vi "VPA QC Calibrate XDCRs.vi"(7 "DAQ Q":T1, 9 "DAQ Ref Cluster":T2, 10 "State Cluster":T4) -> (2 "State Cluster Out":T4)   [LabVIEW 2013]
uses:
  Controls/VPA QC State Data Cluster.ctl
  Controls/VPA QC General Cluster.ctl
  Controls/VPA QC State Enum.ctl
  Controls/VPA QC Bool Cluster.ctl
  Controls/VPA QC DAQ Ref Cluster.ctl
  Controls/VPA QC Scale Communication Settings DVR.ctl
  Controls/VPA QC Scale Communication Settings.ctl
  Controls/VPA QC DAQ Q.ctl
  Controls/VPA QC DAQ Cmd Enum.ctl
panel:
  out "Data Array":dbl[][](array[numeric])
  in  "Take 0 PSI":bool
  in  "Clear Data":bool
  out "Status":string
  out "Best Fit Y-Intercept":dbl format="%0.2f"
  out "Best Fit Slope":dbl format="%0.4f"
  in  "Ramp Down":bool
  in  "Stop Ramp":bool
  out "PcurB":dbl
  in  "Start Ramp":bool
  in  "Pressure Set Point":u32=100 min=100 max=10000
  in  "Open Outlet Valves":bool
  in  "Enterered New\n Volts Constant for B":dbl
  out "Estimated New Max\nVolts for B cylinder.":dbl
  out "PcurA":dbl
  out "A-B Graph":cluster{"X":dbl[], "Y":dbl[]}[](graph)
  in  "Cancel":bool
  in  "Save":bool
  # "Match Pressure Transducers"
  # "Step 1: Make sure the cylinders are initialized and cycled. \nStep 2: Open outlet valves and make sure the cylinders both read 0 psi (or within 1 psi of zero). If they don't zero the transducders."
  # "Step 3: Take a point at 0"
  # "Step 4: Make sure the external outlet valve is closed.\nStep 5. Set the pressue to match the transducers at (you can do this multiple times to see the best fit slope for multiple values.)"
  # "Step 6:"
  # "Monitor the pump. Make sure pump is idle and the external valve is closed. This program will control pressure in a method that bypasses normal procedure.  Turn the pump off if cylinders begin moving too quickly."
  # "Step 7: Determine new volts to use for B side. After ramping pressure down, use terminal to input new max volts for the B cylinder and save the value here for reference."
  # "Suggested\nB Volts"
  # "PcurA"
  # "PcurB"
  # "Dif."
  # "Assembly Checklist"
  # "Assembly Checklist"
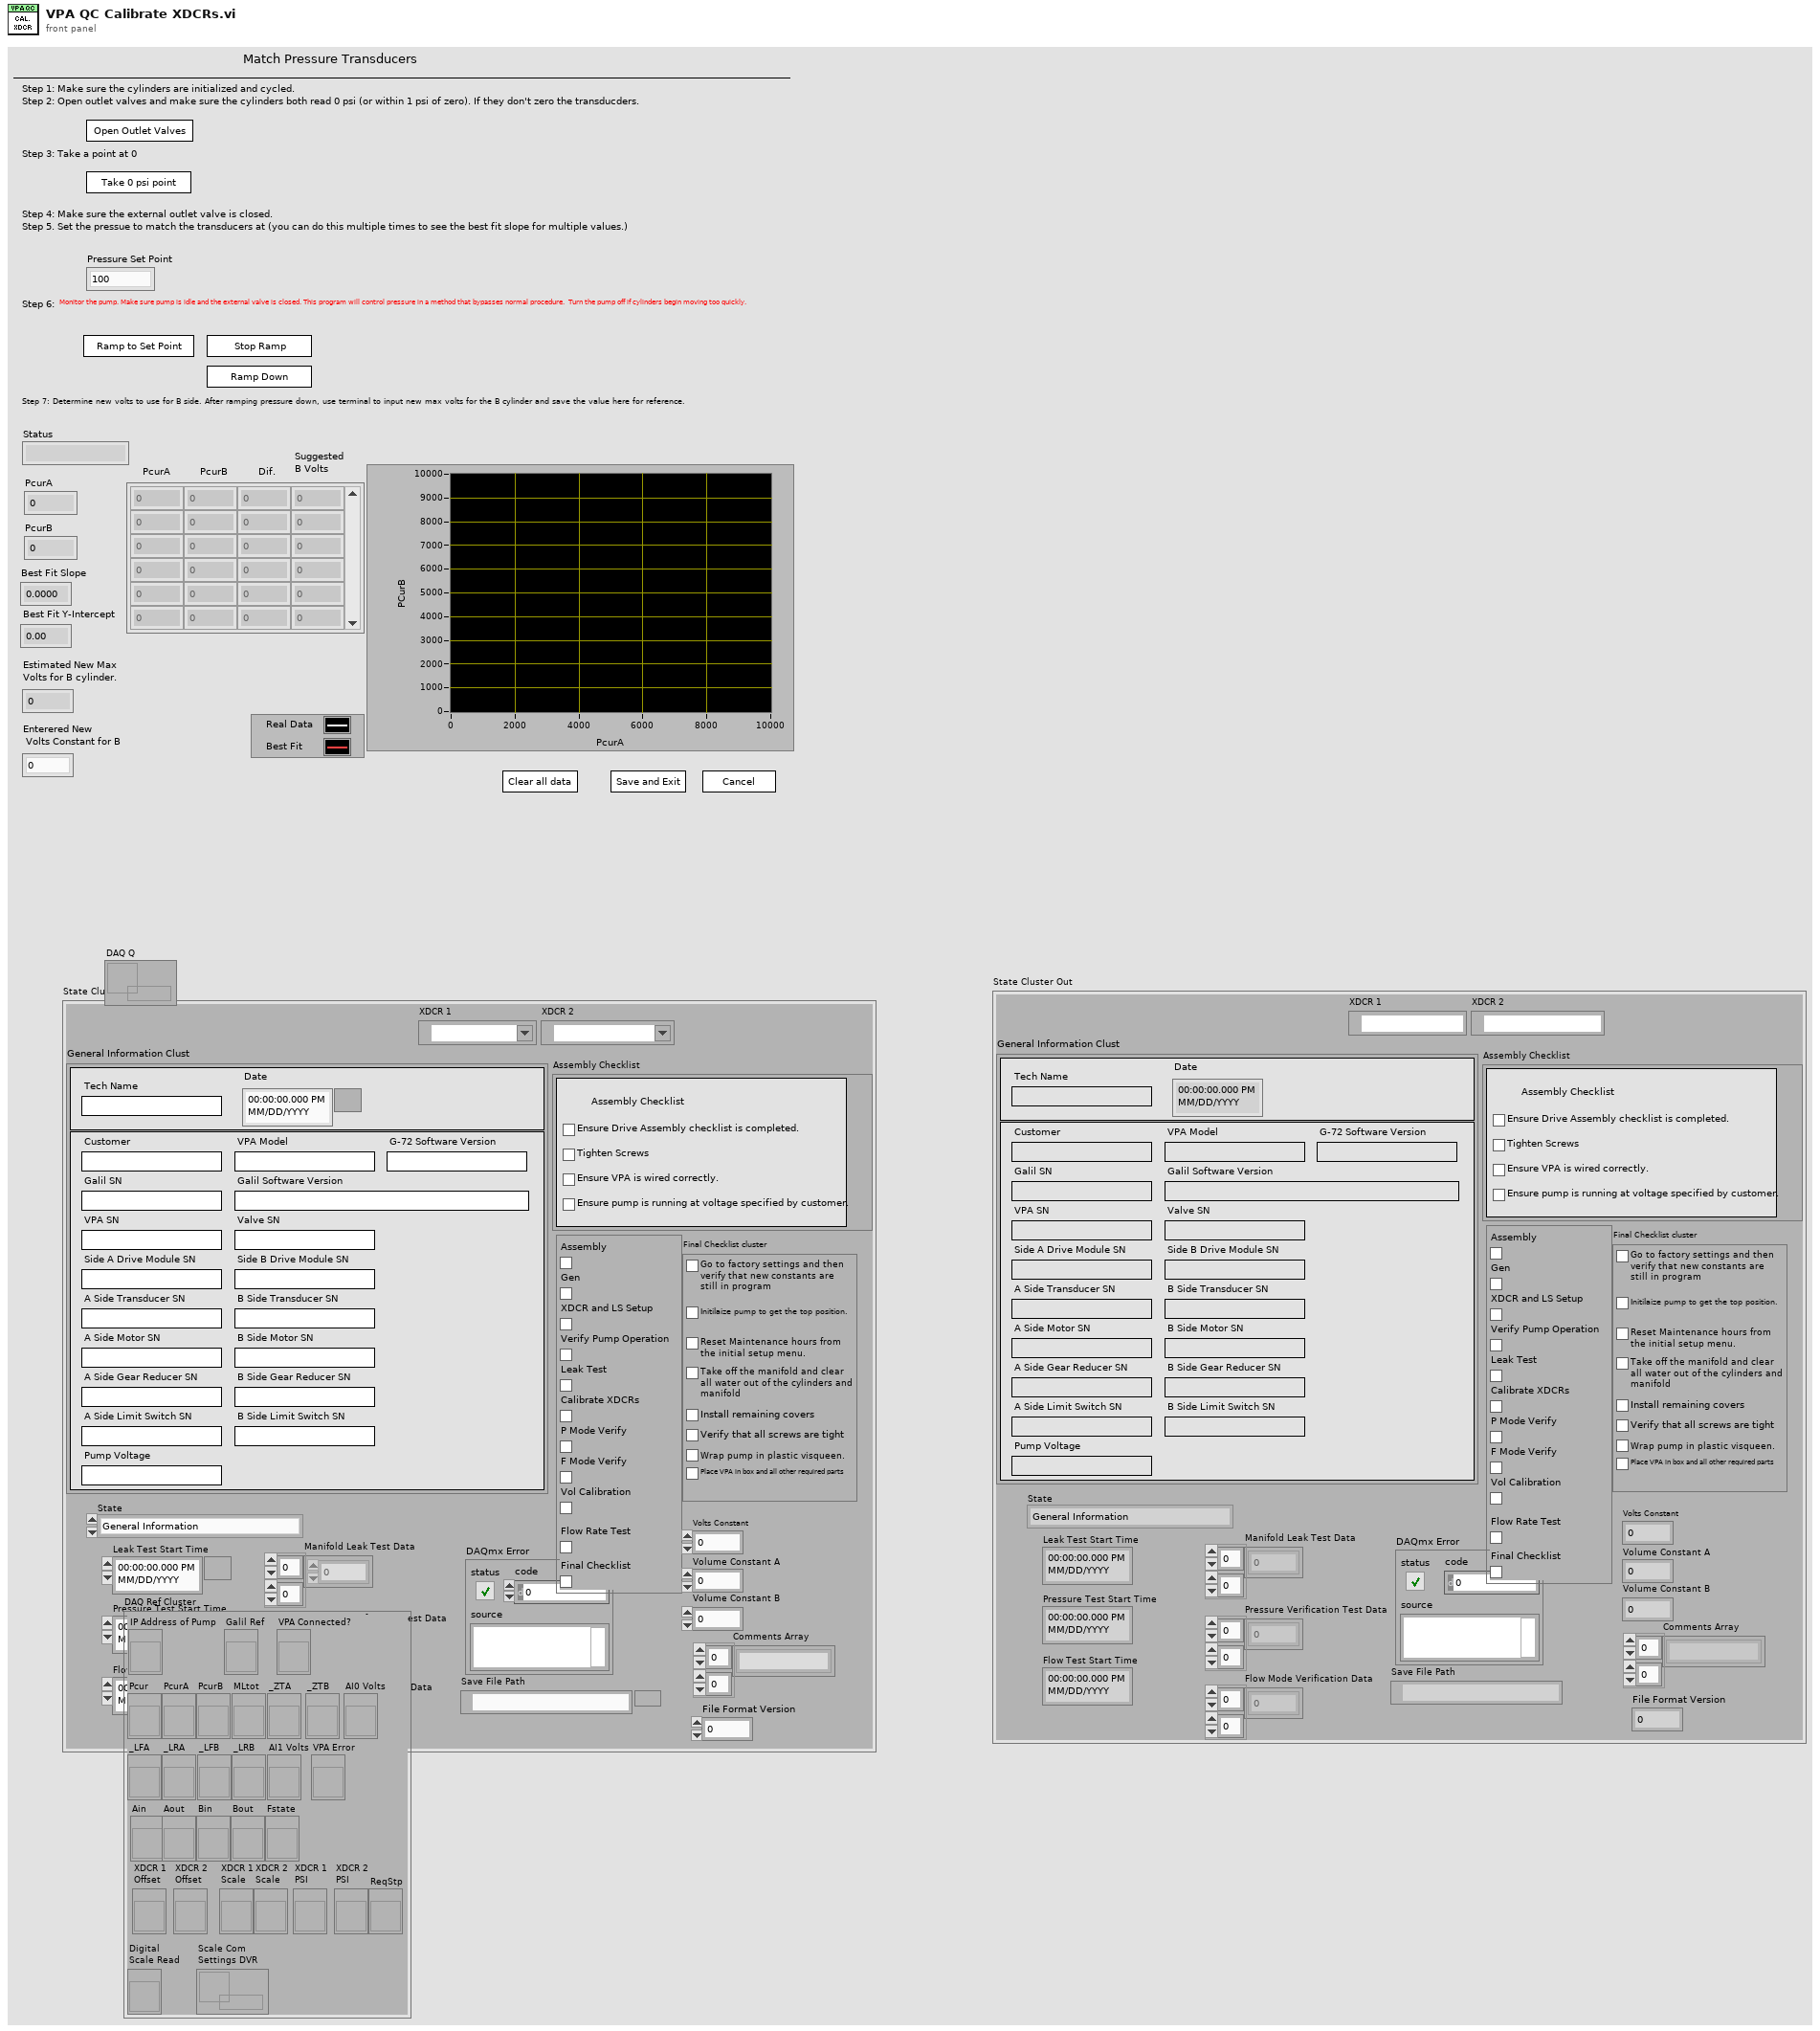
[diagram p1: front panel]
types:
  T1 = typedef "VPA QC DAQ Q.ctl" = refnum<queue>
  T2 = typedef "VPA QC DAQ Ref Cluster.ctl" = cluster{"IP Address of Pump":refnum<vi>, "Galil Ref":refnum<vi>, "VPA Connected?":refnum<vi>, "Pcur":refnum<vi>, "PcurA":refnum<vi>, "PcurB":refnum<vi>, "MLtot":refnum<vi>, "_LFA":refnum<vi>, "_LRA":refnum<vi>, "_LFB":refnum<vi>, "_LRB":refnum<vi>, "_ZTA":refnum<vi>, "_ZTB":refnum<vi>, "AI0 Volts":refnum<vi>, "AI1 Volts":refnum<vi>, "VPA Error":refnum<vi>, "Ain":refnum<vi>, "Aout":refnum<vi>, "Bin":refnum<vi>, "Bout":refnum<vi>, "Fstate":refnum<vi>, "XDCR 1\nOffset":refnum<vi>, "XDCR 2 \nOffset":refnum<vi>, "XDCR 1\nScale":refnum<vi>, "XDCR 2\nScale":refnum<vi>, "XDCR 1\nPSI":refnum<vi>, "XDCR 2\nPSI":refnum<vi>, "ReqStp":refnum<vi>, "Digital \nScale Read":refnum<vi>, "Scale Com\nSettings DVR":T3}
  T3 = typedef "VPA QC Scale Communication Settings DVR.ctl" = refnum<data-value>
  T4 = typedef "VPA QC State Data Cluster.ctl" = cluster{"XDCR 1":tag, "XDCR 2":tag, "General Information Clust":T5, "Assembly Checklist":cluster{"Ensure Drive Assembly checklist is completed.":bool, "Tighten Screws":bool, "Ensure VPA is wired correctly.":bool, "Ensure pump is running at voltage specified by customer.":bool}, "State":T6, "Manifold Leak Test Data":dbl[][], "Pressure Verification Test Data":dbl[][], "Flow Mode Verification Data":dbl[][], "DAQmx Error":errorcluster, "Bool Cluster":T7, "Leak Test Start Time":timestamp, "Pressure Test Start Time":timestamp, "Flow Test Start Time":timestamp, "Final Checklist cluster":cluster{"Check Fact Rest":bool, "Initialize Pump":bool, "Maintenance Hours":bool, "Clean Water Out":bool, "Covers":bool, "Screws":bool, "Wrap":bool, "Box":bool}, "Volts Constant":dbl, "Volume Constant A":dbl, "Volume Constant B":dbl, "Save File Path":path, "Comments Array":string[][], "File Format Version":u16}
  T5 = typedef "VPA QC General Cluster.ctl" = cluster{"Tech Name":string, "Date":timestamp, "Customer":string, "VPA Model":string, "G-72 Software Version":string, "Galil SN":string, "Galil Software Version":string, "VPA SN":string, "Valve SN":string, "Side A Drive Module SN":string, "Side B Drive Module SN":string, "A Side Transducer SN":string, "B Side Transducer SN":string, "A Side Motor SN":string, "B Side Motor SN":string, "A Side Gear Reducer SN":string, "B Side Gear Reducer SN":string, "A Side Limit Switch SN":string, "B Side Limit Switch SN":string, "Pump Voltage":string}
  T6 = typedef "VPA QC State Enum.ctl" = enum16{"General Information", "XDCR and LS Check", "Check Pump Function", "Manifold/Cylinder Leak Test", "Exit"}
  T7 = typedef "VPA QC Bool Cluster.ctl" = cluster{"Assembly":bool, "Gen":bool, "XDCR and LS Setup":bool, "Verify Pump Operation":bool, "Leak Test":bool, "Calibrate XDCRs":bool, "P Mode Verify":bool, "F Mode Verify":bool, "Vol Calibration":bool, "Flow Rate Test":bool, "Final Checklist":bool}
  T8 = enum16{"Idle", "Ramping up", "Ramping down", "Averging data"}
  T9 = typedef "VPA QC DAQ Cmd Enum.ctl" = enum16{"Connect", "Disconnect", "Quit", "Close All Valves", "Burn Calibration", "E-Stop", "Set ZC1", "Set ZC0", "Set ZR", "Open Outlet Valves"}
  T10 = enum8{"Enabled", "Disabled", "Disabled and Grayed Out"}
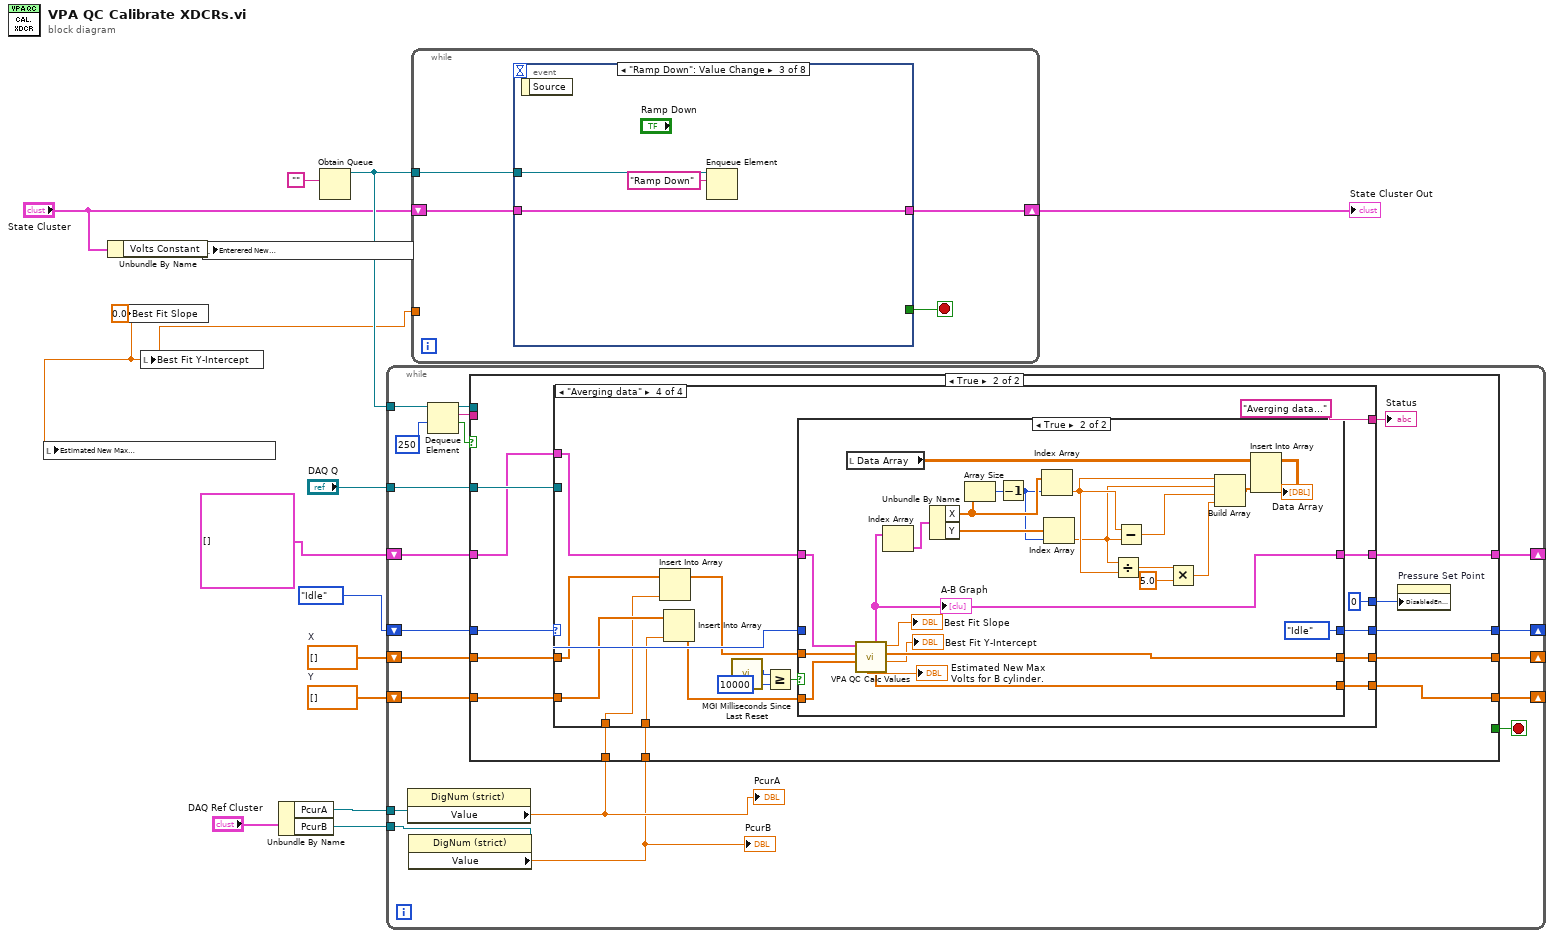
[diagram p0: block diagram]
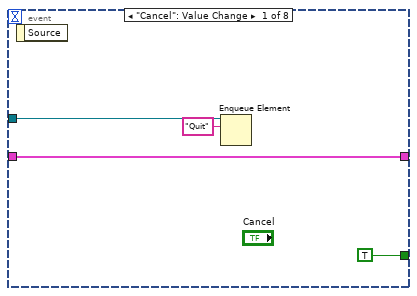
[diagram p2: hidden frame]
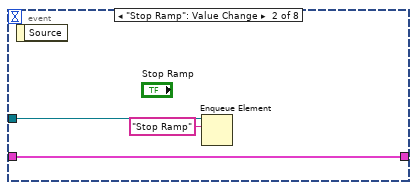
[diagram p3: hidden frame]
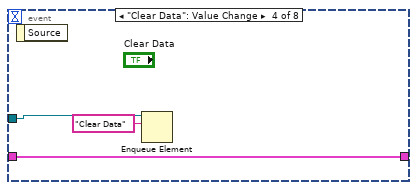
[diagram p4: hidden frame]
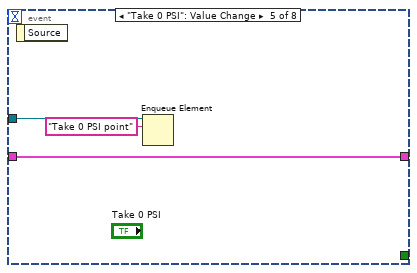
[diagram p5: hidden frame]
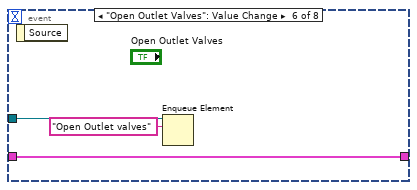
[diagram p6: hidden frame]
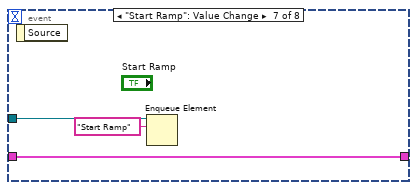
[diagram p7: hidden frame]
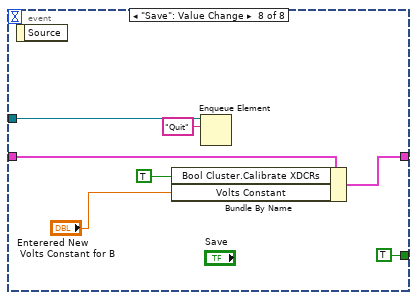
[diagram p8: hidden frame]
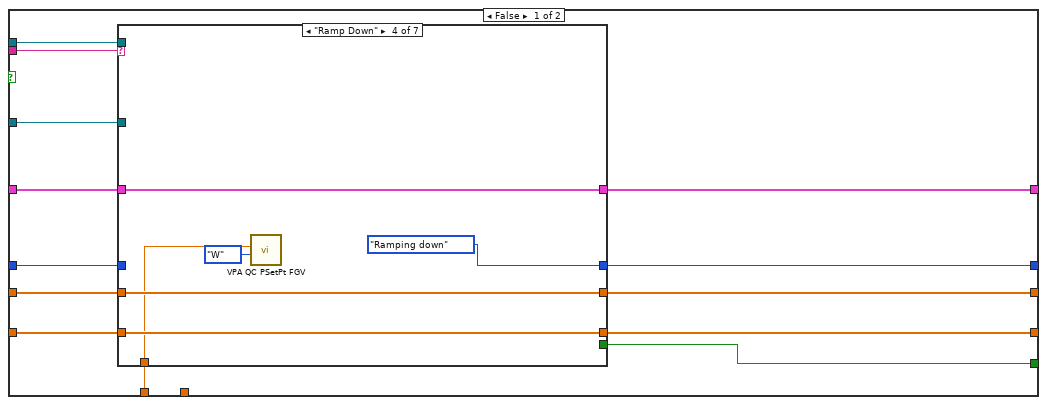
[diagram p9: hidden frame]
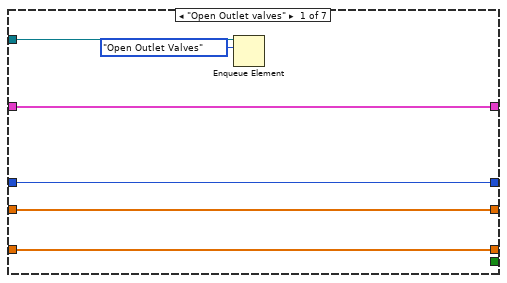
[diagram p10: hidden frame]
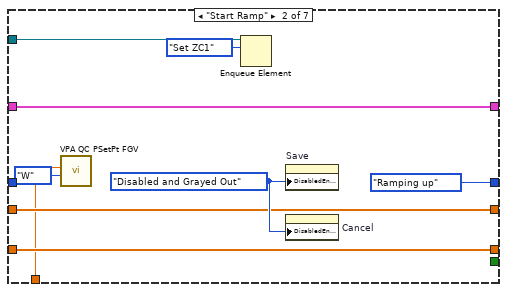
[diagram p11: hidden frame]
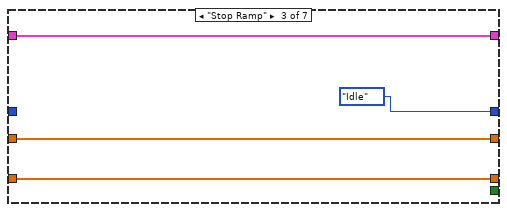
[diagram p12: hidden frame]
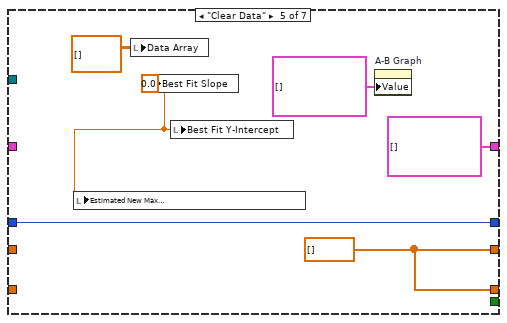
[diagram p13: hidden frame]
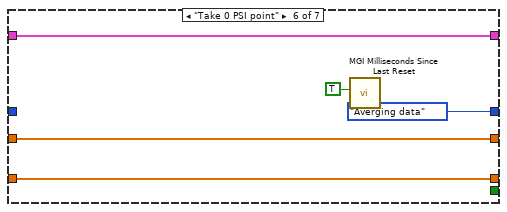
[diagram p14: hidden frame]
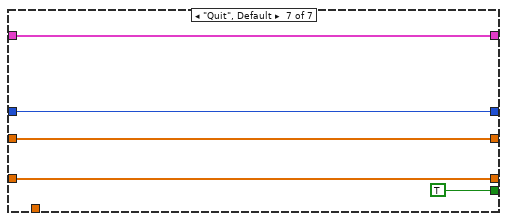
[diagram p15: hidden frame]
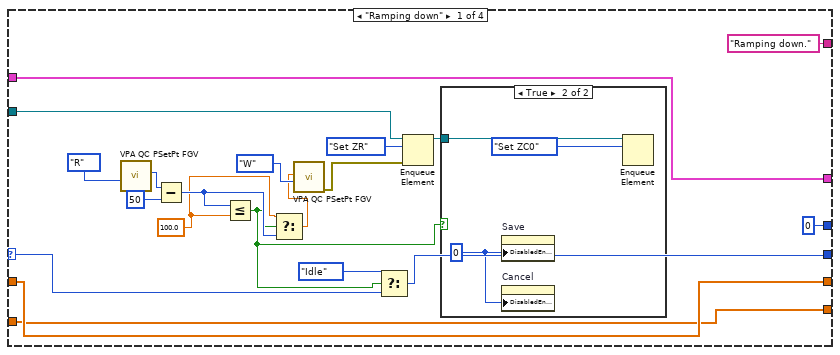
[diagram p16: hidden frame]
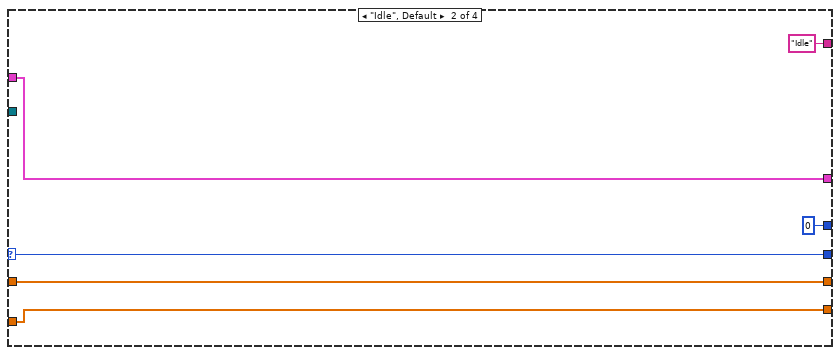
[diagram p18: hidden frame]
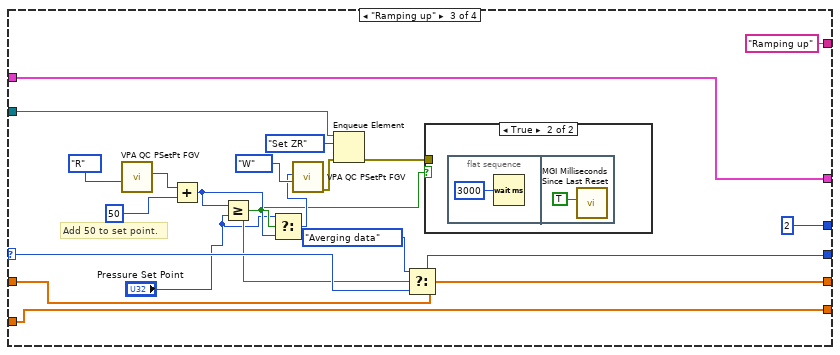
[diagram p19: hidden frame]
diagram:
  w2 = 0.0 ("slope")
  w5 = dbl[] []  # X
  w4 = dbl[] []  # Y
  n1 = local write "Estimated New Max\nVolts for B cylinder."(w2) -> ()
  n2 = Unbundle By Name("State Cluster") -> ("Volts Constant"=w10:dbl)
  n3 = local write "Best Fit Slope"(w2) -> ()
  n4 = local write "Best Fit Y-Intercept"(w2) -> ()
  n5 = local write "Enterered New\n Volts Constant for B"(w10) -> ()
  n6 = Unbundle By Name("DAQ Ref Cluster") -> ("PcurA"=w7:refnum<vi>, "PcurB"=w6:refnum<vi>)
  n7 = Obtain Queue(element data type="") -> (queue out=w13:refnum<queue>)  [unwired: 4 in, 2 out]
  n8 = while {
    tunnel: w13 -> [w33]
    tunnel: "DAQ Q" -> [w28]
    shift-right: [w25] -> _
    shift-left: T8."Idle" ("Testing Phase") -> [w26]
    tunnel: w7 -> [w24]
    tunnel: w6 -> [w23]
    shift-right: [w19] -> _
    shift-left: cluster{"X":dbl[], "Y":dbl[]}[] [] -> [w20]
    shift-right: [w16] -> _
    shift-left: w5 -> [w17]
    shift-right: [w15] -> _
    shift-left: w4 -> [w18]
    stop <- w27 stop-if-true
    n9 = property class="DigNum (strict)"(reference=w24) -> ("Value"=w22:dbl)  [unwired: 1 in, 2 out]
    "PcurA" <- w22
    n10 = property class="DigNum (strict)"(reference=w23) -> ("Value"=w21:dbl)  [unwired: 1 in, 2 out]
    "PcurB" <- w21
    n11 = Dequeue Element(queue=w33, timeout in ms (-1)=250) -> (queue out=w29:refnum<queue>, element=w31:string, timed out?=w30:bool)  [unwired: 1 in, 1 out]
    n12 = case shown="True" w30 {
      tunnel: w31 -> [w46 _]
      tunnel: w29 -> [w43 _]
      tunnel: w28 -> [w44 w100]
      tunnel: [w45 _] -> w27
      tunnel: w26 -> [w42 w99]
      tunnel: [w41 w98] -> w25
      tunnel: w22 -> [w34 w97]
      tunnel: w21 -> [_ w96]
      tunnel: w20 -> [w40 w95]
      tunnel: [w39 w94] -> w19
      tunnel: w18 -> [w36 w92]
      tunnel: w17 -> [w38 w93]
      tunnel: [w37 w91] -> w16
      tunnel: [w35 w90] -> w15
      frame False {
        n13 = case shown="\"Ramp Down\"" w46 {
          tunnel: [_ _ _ _ _ _ TRUE] -> w45
          tunnel: w44 -> [w52 w61 _ _ _ _ _]
          tunnel: w43 -> [_ _ _ _ _ _ _]
          tunnel: w42 -> [w50 _ _ _ w77 _ w86]
          tunnel: [w50 T8."Ramping up" ("Testing Phase") T8."Idle" ("Testing Phase") T8."Ramping down" ("Testing Phase") w77 T8."Averging data" ("Testing Phase") w86] -> w41
          tunnel: w40 -> [w49 w58 w65 w71 _ w82 w85]
          tunnel: [w49 w58 w65 w71 cluster{"X":dbl[], "Y":dbl[]}[] [] w82 w85] -> w39
          tunnel: w38 -> [w48 w57 w64 w70 _ w81 w84]
          tunnel: [w48 w57 w64 w70 w75 w81 w84] -> w37
          tunnel: w36 -> [w47 w56 w63 w69 _ w80 w83]
          tunnel: [w47 w56 w63 w69 w75 w80 w83] -> w35
          tunnel: w34 -> [_ w54 _ w67 _ _ _]
          frame "Open Outlet valves" {
            n14 = Enqueue Element(queue=w52, element=VPA_QC_DAQ_Cmd_Enum."Open Outlet Valves") -> ()  [unwired: 2 in, 3 out]
          }
          frame "Start Ramp" {
            w59 = T10."Disabled and Grayed Out" ("Disabled")
            n15 = call "VPA QC PSetPt FGV.vi"("Function"=enum16{"R", "W"}."W", "PSetPt In"=w54) -> ()  [unwired: 8 in, 2 out]
            n16 = Enqueue Element(queue=w61, element=VPA_QC_DAQ_Cmd_Enum."Set ZC1") -> ()  [unwired: 2 in, 3 out]
            n17 = property on="Save" class="Bool"("DisabledEnum"=w59) -> ()  [unwired: 2 in, 2 out]
            n18 = property on="Cancel" class="Bool"("DisabledEnum"=w59) -> ()  [unwired: 2 in, 2 out]
          }
          frame "Stop Ramp" {
          }
          frame "Ramp Down" {
            n19 = call "VPA QC PSetPt FGV.vi"("Function"=enum16{"R", "W"}."W", "PSetPt In"=w67) -> ()  [unwired: 8 in, 2 out]
          }
          frame "Clear Data" {
            w73 = 0.0 ("slope")
            w75 = dbl[] [] ("X")
            n20 = local write "Estimated New Max\nVolts for B cylinder."(w73) -> ()
            n21 = local write "Data Array"(dbl[][] [] ("Data Array")) -> ()
            n22 = local write "Best Fit Slope"(w73) -> ()
            n23 = local write "Best Fit Y-Intercept"(w73) -> ()
            n24 = property on="A-B Graph" class="XYGraph (strict)"("Value"=cluster{"X":dbl[], "Y":dbl[]}[] [] ("A-B Graph")) -> ()  [unwired: 2 in, 2 out]
          }
          frame "Take 0 PSI point" {
            n25 = call <userlib>:"MGI Milliseconds Since Last Reset.vi"("Reset (F)"=TRUE) -> ()  [unwired: 5 in, 2 out]
          }
          frame "Quit", Default {
          }
        }
      }
      frame True {
        n26 = case shown="\"Averging data\"" w99 {
          selector: w99 -> [w112 w129 w141 w162]
          tunnel: w100 -> [w116 _ w145 _]
          tunnel: [w111 w129 w140 w161] -> w98
          tunnel: w97 -> [_ _ _ w155]
          tunnel: w96 -> [_ _ _ w154]
          tunnel: w95 -> [w108 w128 w139 w160]
          tunnel: [w108 w128 w139 w165] -> w94
          tunnel: w93 -> [w106 w127 w136 w156]
          tunnel: w92 -> [w105 w126 w135 w158]
          tunnel: [w106 w127 w136 w164] -> w91
          tunnel: [w105 w126 w135 w163] -> w90
          tunnel: ["Ramping down." "Idle" "Ramping up" "Averging data..."] -> w89
          tunnel: [0 0 2 0] -> w88
          frame "Ramping down" {
            w107 = 100.0 ("t")
            n27 = call "VPA QC PSetPt FGV.vi"("Function"=enum16{"R", "W"}."R") -> ("PSetPt Out"=w118:u32)  [unwired: 9 in, 1 out]
            n28 = Subtract(x=w118, y=u32 50) -> (x-y=w114:u32)
            n29 = Less Or Equal?(x=w114, y=w107) -> (x <= y?=w110:bool)
            n30 = Select(t=w107, s=w110, f=w114) -> (s? t:f=w113:dbl)
            n31 = call "VPA QC PSetPt FGV.vi"("Function"=enum16{"R", "W"}."W", "PSetPt In"=w113) -> ("error out"=w117:errorcluster)  [unwired: 8 in, 1 out]
            n32 = Select(t=T8."Idle" ("Testing Phase"), s=w110, f=w112) -> (s? t:f=w111:T8)
            n33 = Enqueue Element(queue=w116, element=VPA_QC_DAQ_Cmd_Enum."Set ZR", error in (no error)=w117) -> (queue out=w109:T1)  [unwired: 1 in, 2 out]
            n34 = case shown="True" w110 {
              tunnel: w109 -> [_ w123]
              frame False {
              }
              frame True {
                w121 = 0
                n35 = property on="Save" class="Bool"("DisabledEnum"=w121) -> ()  [unwired: 2 in, 2 out]
                n36 = property on="Cancel" class="Bool"("DisabledEnum"=w121) -> ()  [unwired: 2 in, 2 out]
                n37 = Enqueue Element(queue=w123, element=VPA_QC_DAQ_Cmd_Enum."Set ZC0") -> ()  [unwired: 2 in, 3 out]
              }
            }
          }
          frame "Idle", Default {
          }
          frame "Ramping up" {
            # "Add 50 to set point."
            n38 = call "VPA QC PSetPt FGV.vi"("Function"=enum16{"R", "W"}."R") -> ("PSetPt Out"=w147:u32)  [unwired: 9 in, 1 out]
            n39 = Add(x=w147, y=u32 50) -> (x+y=w143:u32)
            n40 = Greater Or Equal?(x=w143, y="Pressure Set Point") -> (x >= y?=w138:bool)
            n41 = Select(t="Pressure Set Point", s=w138, f=w143) -> (s? t:f=w142:u32)
            n42 = call "VPA QC PSetPt FGV.vi"("Function"=enum16{"R", "W"}."W", "PSetPt In"=w142) -> ("error out"=w146:errorcluster)  [unwired: 8 in, 1 out]
            n43 = Enqueue Element(queue=w145, element=VPA_QC_DAQ_Cmd_Enum."Set ZR", error in (no error)=w146) -> (error out=w131:errorcluster)  [unwired: 1 in, 2 out]
            n44 = Select(t=T8."Averging data" ("Testing Phase"), s=w138, f=w141) -> (s? t:f=w140:T8)
            n45 = case shown="True" w138 {
              tunnel: w131 -> [_ _]
              frame False {
              }
              frame True {
                n46 = flat-sequence {
                  frame #0 {
                    n47 = Wait (ms)(milliseconds to wait=u32 3000 ("millisecond multiple")) -> ()  [unwired: 1 out]
                  }
                  frame #1 {
                    n48 = call <userlib>:"MGI Milliseconds Since Last Reset.vi"("Reset (F)"=TRUE) -> ()  [unwired: 5 in, 2 out]
                  }
                }
              }
            }
          }
          frame "Averging data" {
            n49 = Insert Into Array(array=w156, new element=w155) -> (w159:dbl[])  [unwired: 1 in]
            n50 = Insert Into Array(array=w158, new element=w154) -> (w157:dbl[])  [unwired: 1 in]
            n51 = call <userlib>:"MGI Milliseconds Since Last Reset.vi"() -> ("ms"=w168:u32)  [unwired: 6 in, 1 out]
            n52 = Greater Or Equal?(x=w168, y=u32 10000) -> (x >= y?=w166:bool)
            n53 = case shown="True" w166 {
              tunnel: w160 -> [w172 w192]
              tunnel: [w172 w187] -> w165
              tunnel: [w171 w195] -> w164
              tunnel: [w170 w194] -> w163
              tunnel: w159 -> [w171 w191]
              tunnel: w157 -> [w170 w193]
              tunnel: w162 -> [w169 _]
              tunnel: [w169 T8."Idle" ("Testing Phase")] -> w161
              frame False {
                # "Not done getting 10 seconds of samples"
              }
              frame True {
                n54 = local read "Data Array"() -> (w179:dbl[][])
                n55 = call "VPA QC Calc Values.vi"("Y in"=w193, "X in"=w191, "Array in"=w192) -> ("intercept"=→"Best Fit Y-Intercept":dbl, "X out"=w195:dbl[], "slope"=→"Best Fit Slope":dbl, "Y out"=w194:dbl[], "Array out"=w187:cluster{"X":dbl[], "Y":dbl[]}[], "Suggested Volts"=→"Estimated New Max\nVolts for B cylinder.":dbl)  [unwired: 3 in]
                "A-B Graph" <- w187
                n56 = Index Array(array=w187) -> (element=w186:cluster{"X":dbl[], "Y":dbl[]})  [unwired: 1 in]
                n57 = Unbundle By Name(w186) -> ("X"=w184:dbl[], "Y"=w183:dbl[])
                n58 = Array Size(array=w184) -> (size(s)=w185:i32)
                n59 = Decrement(x=w185) -> (x-1=w173:i32)
                n60 = Index Array(array=w184, index=w173) -> (element=w182:dbl)
                n61 = Index Array(array=w183, index=w173) -> (element=w181:dbl)
                n62 = Divide(x=w181, y=w182) -> (x/y=w176:dbl)
                n63 = Subtract(x=w182, y=w181) -> (x-y=w180:dbl)
                n64 = Multiply(x=w176, y=5.0) -> (x*y=w174:dbl)
                n65 = Build Array(w182, w181, w180, w174) -> (w177:dbl[])
                n66 = Insert Into Array(array=w179, new element=w177) -> (→"Data Array":dbl[][])  [unwired: 2 in]
              }
            }
          }
        }
        "Status" <- w89
        n67 = property on="Pressure Set Point" class="DigNum (strict)"("DisabledEnum"=w88) -> ()  [unwired: 2 in, 2 out]
      }
    }
  }
  n68 = while {
    tunnel: w13 -> [w199]
    shift-right: [w197] -> w12
    shift-left: "State Cluster" -> [w198]
    tunnel: w2 -> [_]
    stop <- w200 stop-if-true
    n69 = event shown="[2] \"Ramp Down\": Value Change" {
      selector: _ -> [_ _ _ _ _ _ _ _]
      dyn-events: _ -> [_ _ _ _ _ _ _ _]
      timeout: _ -> [_ _ _ _ _ _ _ _]
      tunnel: [TRUE _ _ _ _ _ _ TRUE] -> w200
      tunnel: w199 -> [w203 w206 w209 w212 w215 w218 w221 w225]
      tunnel: w198 -> [w201 w207 w210 w213 w216 w219 w222 w228]
      tunnel: [w201 w207 w210 w213 w216 w219 w222 w226] -> w197
      event "Cancel": Value Change {
        n70 = event-data() -> ()  [unwired: 1 in, 1 out]
        n71 = Enqueue Element(queue=w203, element="Quit") -> ()  [unwired: 2 in, 3 out]
      }
      event "Stop Ramp": Value Change {
        n72 = event-data() -> ()  [unwired: 1 in, 1 out]
        n73 = Enqueue Element(queue=w206, element="Stop Ramp") -> ()  [unwired: 2 in, 3 out]
      }
      event "Ramp Down": Value Change {
        n74 = event-data() -> ()  [unwired: 1 in, 1 out]
        n75 = Enqueue Element(queue=w209, element="Ramp Down") -> ()  [unwired: 2 in, 3 out]
      }
      event "Clear Data": Value Change {
        n76 = event-data() -> ()  [unwired: 1 in, 1 out]
        n77 = Enqueue Element(queue=w212, element="Clear Data") -> ()  [unwired: 2 in, 3 out]
      }
      event "Take 0 PSI": Value Change {
        n78 = event-data() -> ()  [unwired: 1 in, 1 out]
        n79 = Enqueue Element(queue=w215, element="Take 0 PSI point") -> ()  [unwired: 2 in, 3 out]
      }
      event "Open Outlet Valves": Value Change {
        n80 = event-data() -> ()  [unwired: 1 in, 1 out]
        n81 = Enqueue Element(queue=w218, element="Open Outlet valves") -> ()  [unwired: 2 in, 3 out]
      }
      event "Start Ramp": Value Change {
        n82 = event-data() -> ()  [unwired: 1 in, 1 out]
        n83 = Enqueue Element(queue=w221, element="Start Ramp") -> ()  [unwired: 2 in, 3 out]
      }
      event "Save": Value Change {
        n84 = event-data() -> ()  [unwired: 1 in, 1 out]
        n85 = Bundle By Name(cluster=w228, "Bool Cluster.Calibrate XDCRs"=TRUE ("Bool Cluster.Leak Test"), "Volts Constant"="Enterered New\n Volts Constant for B") -> (w226:T4)
        n86 = Enqueue Element(queue=w225, element="Quit") -> ()  [unwired: 2 in, 3 out]
      }
    }
  }
  "State Cluster Out" <- w12
